vi "PanelToJSON.vi"(8 "error in (no error)":errorcluster, 9 "Owner Bounds":T1, 10 "Controls[]":refnum<vi>[](array[refnum]), 11 "Folder Path":path) -> (0 "error out":errorcluster, 2 "spreadsheet string":string)   [LabVIEW 2017]
uses:
  <vilib>/Utility/miscctls.llb/LVRectTypeDef.ctl
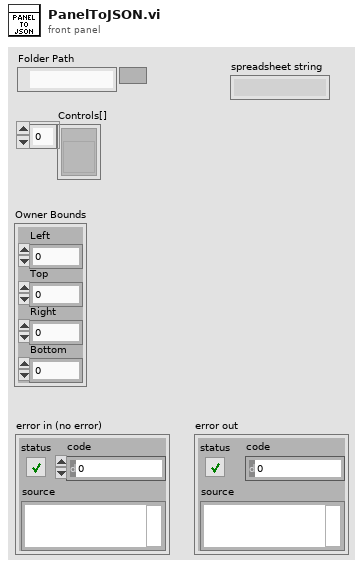
[diagram p1: front panel]
types:
  T1 = typedef "LVRectTypeDef.ctl" = cluster{"Left":i16, "Top":i16, "Right":i16, "Bottom":i16}
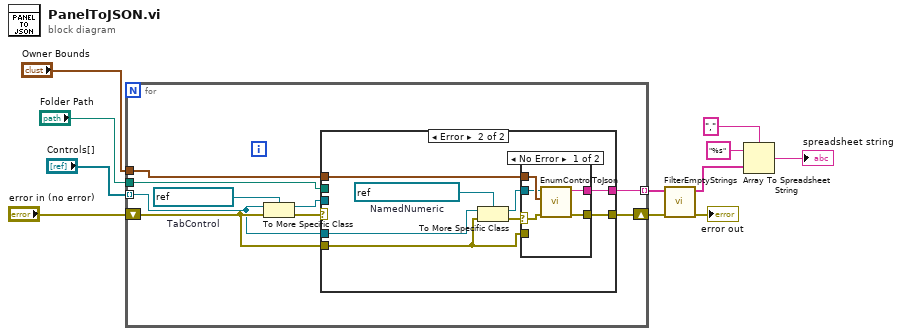
[diagram p0: block diagram]
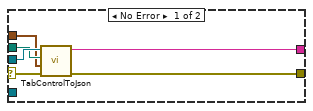
[diagram p2: hidden frame]
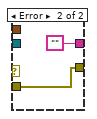
[diagram p3: hidden frame]
diagram:
  n1 = for {
    tunnel: "Controls[]" -> [w13] mode=indexing
    tunnel: "Folder Path" -> [w18]
    tunnel: [w17] -> w6 mode=indexing
    shift-right: [w15] -> w3
    shift-left: "error in (no error)" -> [w14]
    tunnel: "Owner Bounds" -> [w12]
    w20 = refnum<vi> refnum  # TabControl
    n2 = To More Specific Class(target class=w20, reference=w13, error in=w14) -> (specific class reference=w19:refnum<vi>, error out=w16:errorcluster)
    n3 = case shown="Error" w16 {
      selector: w16 -> [w22 _]
      tunnel: w19 -> [w26 _]
      tunnel: w18 -> [w25 _]
      tunnel: [w24 w30] -> w15
      tunnel: [w23 w27] -> w17
      tunnel: w14 -> [_ w28]
      tunnel: w13 -> [_ w34]
      tunnel: w12 -> [w21 w32]
      frame No Error {
        n4 = call "TabControlToJson.vi"("error in (no error)"=w22, "Owner Bounds"=w21, "Folder Path"=w25, "TabControl in"=w26) -> ("error out"=w24:errorcluster, "String out"=w23:string)  [unwired: 6 in]
      }
      frame Error {
        w33 = refnum<vi> refnum  # NamedNumeric
        n5 = To More Specific Class(target class=w33, reference=w34, error in=w28) -> (specific class reference=w31:refnum<vi>, error out=w29:errorcluster)
        n6 = case shown="No Error" w29 {
          selector: w29 -> [w36 _]
          tunnel: w32 -> [w39 _]
          tunnel: w31 -> [w38 _]
          tunnel: [w37 w41] -> w30
          tunnel: w28 -> [_ w41]
          tunnel: [w35 ""] -> w27
          frame No Error {
            n7 = call "EnumControlToJson.vi"("error in (no error)"=w36, "Owner Bounds"=w39, "NamedNumeric in"=w38) -> ("error out"=w37:errorcluster, "String"=w35:string)  [unwired: 7 in]
          }
          frame Error {
          }
        }
      }
    }
  }
  n8 = call "FilterEmptyStrings.vi"("error in"=w3, "Array in"=w6) -> ("error out"=→"error out":errorcluster, "Array out"=w5:string[])  [unwired: 8 in]
  n9 = Array To Spreadsheet String(delimiter (Tab)=",", array=w5, 3:"%s" ("format string")) -> (spreadsheet string=→"spreadsheet string":string)
